vi "Telescope Close.vi"(8 "error in (no error)":errorcluster, 11 "PRIME Telescope in":refnum<class "PRIME Telescope.lvclass">) -> (0 "error out":errorcluster, 3 "PRIME Telescope out":refnum<class "PRIME Telescope.lvclass">)   [LabVIEW 2024, in "PRIME Telescope.lvclass"]
uses:
  PRIME Telescope.lvclass
  PRIME Telescope.lvclass/PRIME Telescope.ctl
  Telescope.lvclass
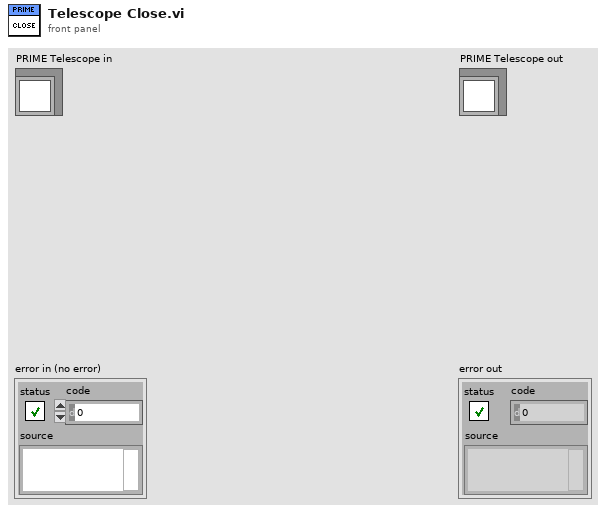
[diagram p1: front panel]
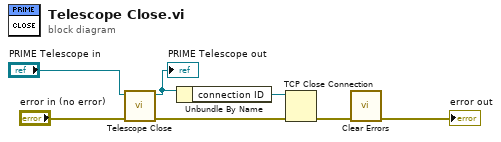
[diagram p0: block diagram]
diagram:
  n1 = call-parent "Telescope Close.vi"("error in (no error)"="error in (no error)", "Telescope in"="PRIME Telescope in") -> ("error out"=w3:errorcluster, "Telescope out"=w5:refnum<class "PRIME Telescope.lvclass">)  [unwired: 8 in]
  "PRIME Telescope out" <- w5
  n2 = Unbundle By Name(w5) -> ("connection ID"=w4:refnum<k5>)
  n3 = TCP Close Connection(connection ID=w4, error in (no error)=w3) -> (error out=w2:errorcluster)  [unwired: 1 in, 1 out]
  n4 = call <vilib>:"Clear Errors.vi"("error in (no error)"=w2) -> ("error out"=→"error out":errorcluster)  [unwired: 5 in, 1 out]
